vi "Get 2D CXT.vi"(5 "format string (%_20f)":string="%_20f", 7 "key description":string, 8 "sections":string[](array[string]), 9 "numeric":cxt[][](array[numeric]), 11 "info data":string) -> (0 "sections out":string[](array[string]), 1 "key found?":bool, 2 "value":cxt[][](array[numeric]) format="%.2f", 3 "info data out":string)   [LabVIEW 2013, in "infolib.lvlib"]
doc: "Add a new numeric key to Info Data string. If section exists in Info Data string, inserts key into this section."
uses:
  infolib.lvlib
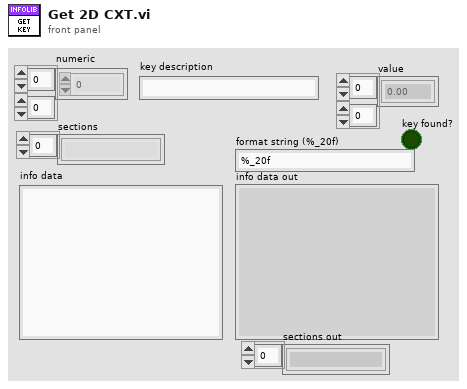
[diagram p1: front panel]
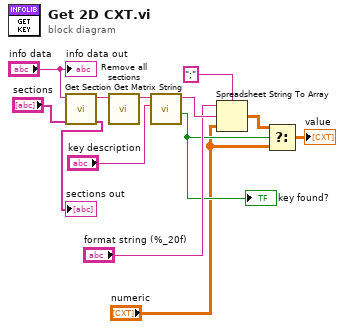
[diagram p0: block diagram]
diagram:
  n1 = call "Get Section.vi"("sections"="sections", "info data"="info data") -> ("sections out"=→"sections out":string[], "section part"=w13:string)  [unwired: 7 in, 1 out]
  n2 = call "Remove all sections.vi"("info data"=w13) -> ("info data out"=w11:string)  [unwired: 10 in]
  n3 = call "Get Matrix String.vi"("matrix key"="key description", "info data"=w11) -> ("key found?"=w3:bool, "matrix part"=w9:string)  [unwired: 8 in]
  "key found?" <- w3
  n4 = Spreadsheet String To Array(delimiter (Tab)=";", format string="format string (%_20f)", spreadsheet string=w9, array type (2D Dbl)="numeric") -> (array=w4:cxt[][])
  n5 = Select(t=w4, s=w3, f="numeric") -> (s? t:f=→"value":cxt[][])
  "info data out" <- "info data"
